vi "SSC Digital PPMU Configure Voltage Limits.vi"(0 "Digital SSC in":T1[](array[typedef]), 5 "Voltage Limit High (V)":dbl=2.5 format="%#_13g", 7 "Voltage Limit Low (V)":dbl=-1.5 format="%#_13g", 11 "error in":errorcluster) -> (4 "Digital SSC out":T1[](array[typedef]), 15 "error out":errorcluster)   [LabVIEW 2020]
doc: "Specifies the voltage limit high, or high clamp voltage (VCH), and voltage limit low, or low clamp voltage (VCL) for the specified pins and pin group(s) when forcing current. You must call the PPMU Source VI for changes to the PPMU configuration to take effect, even if the PPMU is already sourcing."
uses:
  SSC Digital.ctl
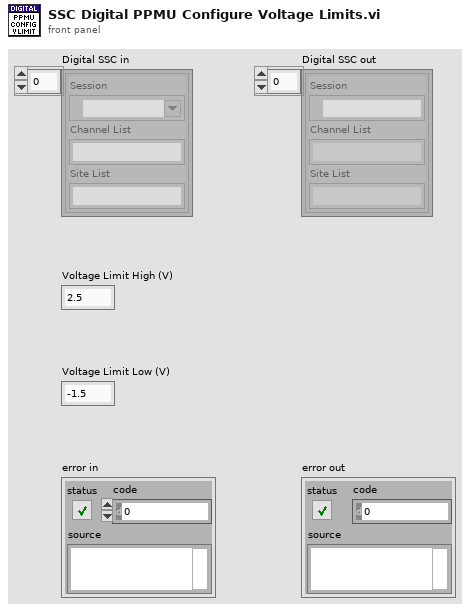
[diagram p1: front panel]
types:
  T1 = typedef "SSC Digital.ctl" = cluster{"Session":refnum<k15>, "Channel List":string, "Site List":string}
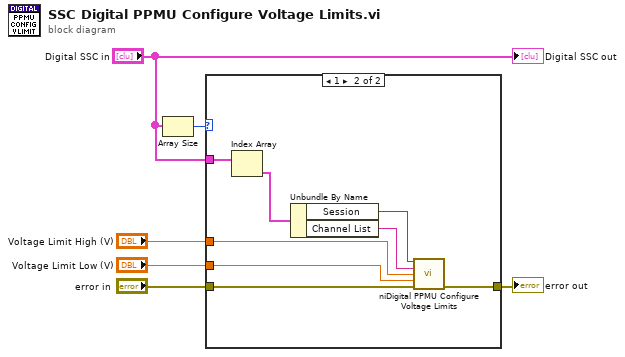
[diagram p0: block diagram]
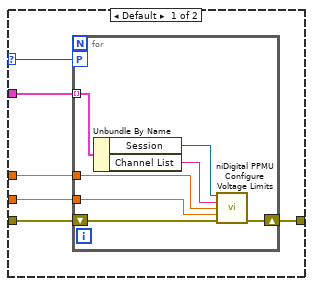
[diagram p2: hidden frame]
diagram:
  n1 = Array Size(array="Digital SSC in") -> (size(s)=w2:i32)
  n2 = case shown="1" w2 {
    selector: w2 -> [w8 _]
    tunnel: "Voltage Limit High (V)" -> [w12 w27]
    tunnel: "Voltage Limit Low (V)" -> [w11 w26]
    tunnel: "error in" -> [w10 w25]
    tunnel: [w9 w24] -> w3
    tunnel: "Digital SSC in" -> [w7 w23]
    frame Default {
      n3 = for {
        tunnel: w12 -> [w18]
        tunnel: w11 -> [w17]
        workers-P: w8 -> [_]
        tunnel: w7 -> [w14] mode=indexing
        shift-right: [w13] -> w9
        shift-left: w10 -> [w19]
        n4 = Unbundle By Name(w14) -> ("Session"=w15:refnum<k15>, "Channel List"=w16:string)
        n5 = call <instrlib>:"niDigital PPMU Configure Voltage Limits.vi"("instrument handle"=w15, "channel list"=w16, "voltage limit high (V)"=w18, "voltage limit low (V)"=w17, "error in"=w19) -> ("error out"=w13:errorcluster)  [unwired: 9 in, 1 out]
      }
    }
    frame 1 {
      n6 = Index Array(array=w23) -> (element=w20:T1)  [unwired: 1 in]
      n7 = Unbundle By Name(w20) -> ("Session"=w21:refnum<k15>, "Channel List"=w22:string)
      n8 = call <instrlib>:"niDigital PPMU Configure Voltage Limits.vi"("instrument handle"=w21, "channel list"=w22, "voltage limit high (V)"=w27, "voltage limit low (V)"=w26, "error in"=w25) -> ("error out"=w24:errorcluster)  [unwired: 9 in, 1 out]
    }
  }
  "error out" <- w3
  "Digital SSC out" <- "Digital SSC in"
